vi "PH_gentec_M-Link.set Default Settings.vi"(0 "i ref in":refnum<vi>, 5 "error in":errorcluster) -> (14 "i ref out":refnum<vi>, 19 "error out":errorcluster)   [LabVIEW 2014]
doc: "This VI sets Default Settings to wanted Device Settings at own attreibutes. This VI must be placed before the creation of the Proc Events in order to be able to overwrite these later by a Start GOG ..."
uses:
  PH_gentec_M-Link.lvlib
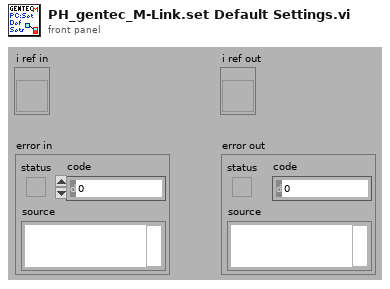
[diagram p1: front panel]
types:
  T1 = typedef "PH_gentec_M-Link.lvlib/PH_gentec_M-Link.i attribute.ctl" = cluster{"GUI References":cluster{"Status":refnum<vi>, "Status Bar":refnum<vi>, "Head Attributes":refnum<vi>, "Wanted Head Settings":refnum<vi>, "Current Head Settings":refnum<vi>, "unscaled Energy [J]":refnum<vi>, "Energy [J]":refnum<vi>, "Energy evolution":refnum<vi>, "Set Auto Range":refnum<vi>, "Range":refnum<vi>, "Trigger Level [%]":refnum<vi>, "Trigger Polarity":refnum<vi>, "Trigger Source":refnum<vi>, "Waveform Averages":refnum<vi>, "Wavelength [nm]":refnum<vi>, "Continuous":refnum<vi>, "Scaling Factor":refnum<vi>, "Connection":refnum<vi>, "Sets 2 change?":refnum<vi>, "get one Value":refnum<vi>}, "Constructor finished?":bool, "Connection":T2, "Head Attributes":T3, "Wanted Head Settings":T6, "Current Head Settings":T6, "Scaling Factor":dbl, "Energy [J]":dbl, "Settings to change?":bool}
  T2 = typedef "PH_gentec_M-Link.lvlib/PH_gentec_M-Link.Connection.ctl" = cluster{"opened":bool, "checked":bool, "failed checks":i8, "Info available":bool, "Timeout":bool, "Data read":string, "Failure":bool, "Error":bool}
  T3 = typedef "PH_gentec_M-Link.lvlib/PH_gentec_M-Link.Head Attributes.ctl" = cluster{"Instrument Type":string, "Head Version":string, "Head Name":string, "Serial Number":string, "Firmware":string, "Sensor Type":T4, "Minimum Range":T5, "Maximum Range":T5, "Minimum Lambda [nm]":i32, "Maximum Lambda [nm]":i32}
  T4 = typedef "gentec-M-LINK.lvlib/gentec-M-Link.Sensor Type.ctl" = u16
  T5 = typedef "gentec-M-LINK.lvlib/gentec-M-Link.Range.ctl" = u16
  T6 = typedef "PH_gentec_M-Link.lvlib/PH_gentec_M-Link.Head Settings.ctl" = cluster{"Measurement Mode":T7, "Enable Anticipation":bool, "Set Auto Range":bool, "Block Signal":bool, "Set Head Attenuator":bool, "Range":T5, "Enable SSE":bool, "Trigger Level [%]":dbl, "Trigger Polarity":T8, "Trigger Source":T9, "Waveform Averages":T10, "Wavelength [nm]":u16, "Set Zero":i32, "Current Measurement":i32, "Start Data Flow":bool}
  T7 = typedef "gentec-M-LINK.lvlib/gentec-M-Link.Measurement Mode.ctl" = u16
  T8 = typedef "gentec-M-LINK.lvlib/gentec-M-Link.Trigger Polarity.ctl" = u16
  T9 = typedef "gentec-M-LINK.lvlib/gentec-M-Link.Trigger Source.ctl" = u16
  T10 = typedef "gentec-M-LINK.lvlib/gentec-M-Link.Waveform Averages.ctl" = u16
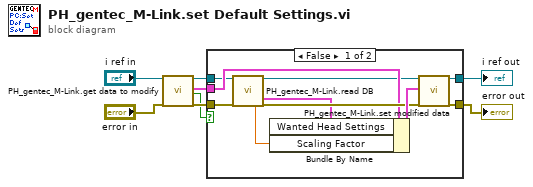
[diagram p0: block diagram]
diagram:
  n1 = call "PH_gentec_M-Link.get data to modify.vi"("i ref in"="i ref in", "error in (no error)"="error in") -> ("i ref out"=w6:refnum<vi>, "i attribute"=w4:T1, "timed out"=w3:bool, "error out"=w5:errorcluster)  [unwired: 14 in]
  n2 = case shown="False" w3 {
    tunnel: [w10 w19] -> w8
    tunnel: [w11 w20] -> w7
    tunnel: w5 -> [w17 w19]
    tunnel: w6 -> [w13 w20]
    tunnel: w4 -> [w15 _]
    frame False {
      n3 = call "PH_gentec_M-Link.read DB.vi"("i ref in"=w13, "error in"=w17) -> ("Default scaling Factor"=w14:dbl, "i ref out"=w12:refnum<vi>, "Default Head Settings"=w9:T6, "error out"=w16:errorcluster)  [unwired: 12 in, 2 out]
      n4 = Bundle By Name(cluster=w15, "Wanted Head Settings"=w9, "Scaling Factor"=w14) -> (w18:T1)
      n5 = call "PH_gentec_M-Link.set modified data.vi"("i ref in"=w12, "i attribute"=w18, "error in (no error)"=w16) -> ("i ref out"=w11:refnum<vi>, "error out"=w10:errorcluster)  [unwired: 15 in]
    }
    frame True {
    }
  }
  "error out" <- w8
  "i ref out" <- w7
